vi "Neutral_ScanAgilentTrim_20151209.vi"(8 "error in (no error)":errorcluster={"status"=FALSE, "code"=0, "source"="gettemp.vi: No error - function call successful"}, 9 "Control Reference Cluster Input":T3, 11 "Triggered Voltage Settings":T1={"Trigger \nDelay (s)"=0.0, "Enable +6V Channel"=FALSE, "+6V Current"=1.0, "Enable -25V Channel"=FALSE, "-25V Current"=0.0, "Enable +25V Channel"=FALSE, "+25V Current"=0.0, "Agilent Rewrite each Cycle"=FALSE} {"Trigger \nDelay (s)" min=0.0 max=3600.0 step=1.0 format="%.2f"}) -> (0 "Error Out":errorcluster)   [LabVIEW 2016]
uses:
  Controls/Agilent E3631A/Settings_Control.ctl
  Controls/Agilent E3631A/Trigger_Settings.ctl
panel:
  in  "Agilent E3631A Settings":T2={"VISA resource name"="GPIB0::5::INSTR", "Voltage Set (6V max)"=6.0, "Current Set (5A max)"=0.007, "Voltage Set (25V max)"=25.0, "Current Set (1A max)"=0.225, "Voltage Set (-25V max)"=25.0, "Current Set (1A max)"=0.225, "6V Switch"=FALSE, "+25V Switch"=FALSE, "-25V Switch"=FALSE} {"Current Set (1A max)" format="%.3g"; "Voltage Set (-25V max)" format="%.3g"; "Current Set (1A max)" format="%.3g"; "Voltage Set (25V max)" format="%.3g"; "Current Set (5A max)" format="%.3g"; "Voltage Set (6V max)" format="%.3g"}
  # "I am assuming here that we will leave the voltage at the maximum and set set the trim field by the current limit. Assuming this will use the voltage settings from the inital programming and only vary the current limit."
  # "-25V Output Settings"
  # "+25V Output Settings"
  # "6V Output Settings"
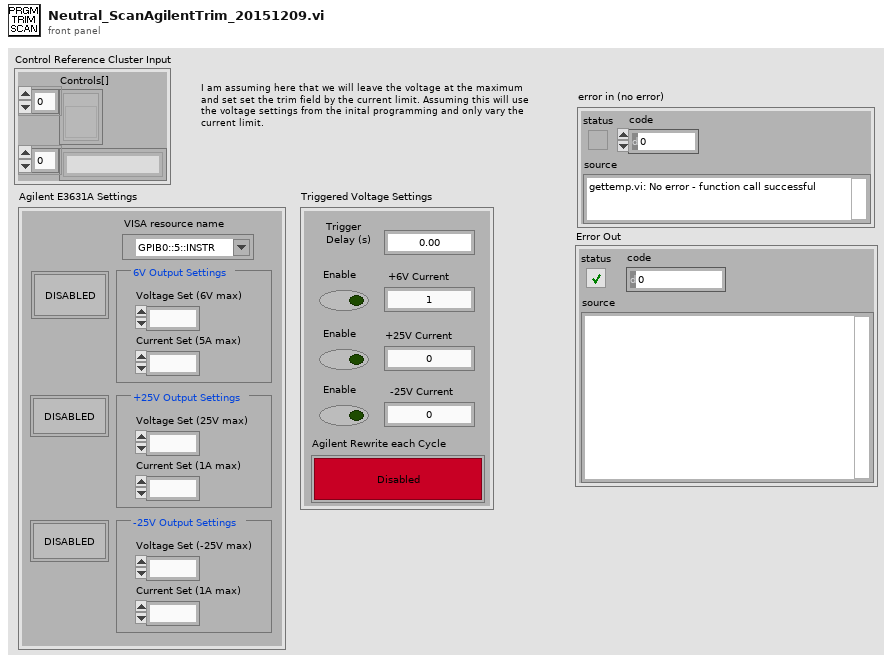
[diagram p1: front panel]
types:
  T1 = typedef "Trigger_Settings.ctl" = cluster{"Trigger \nDelay (s)":dbl, "Enable +6V Channel":bool, "+6V Current":dbl, "Enable -25V Channel":bool, "-25V Current":dbl, "Enable +25V Channel":bool, "+25V Current":dbl, "Agilent Rewrite each Cycle":bool}
  T2 = typedef "Settings_Control.ctl" = cluster{"VISA resource name":refnum<visa-resource-name>, "Voltage Set (6V max)":dbl, "Current Set (5A max)":dbl, "Voltage Set (25V max)":dbl, "Current Set (1A max)":dbl, "Voltage Set (-25V max)":dbl, "Current Set (1A max)":dbl, "6V Switch":bool, "+25V Switch":bool, "-25V Switch":bool}
  T3 = cluster{"Controls[]":refnum<vi>[], "Control Names":string[]}
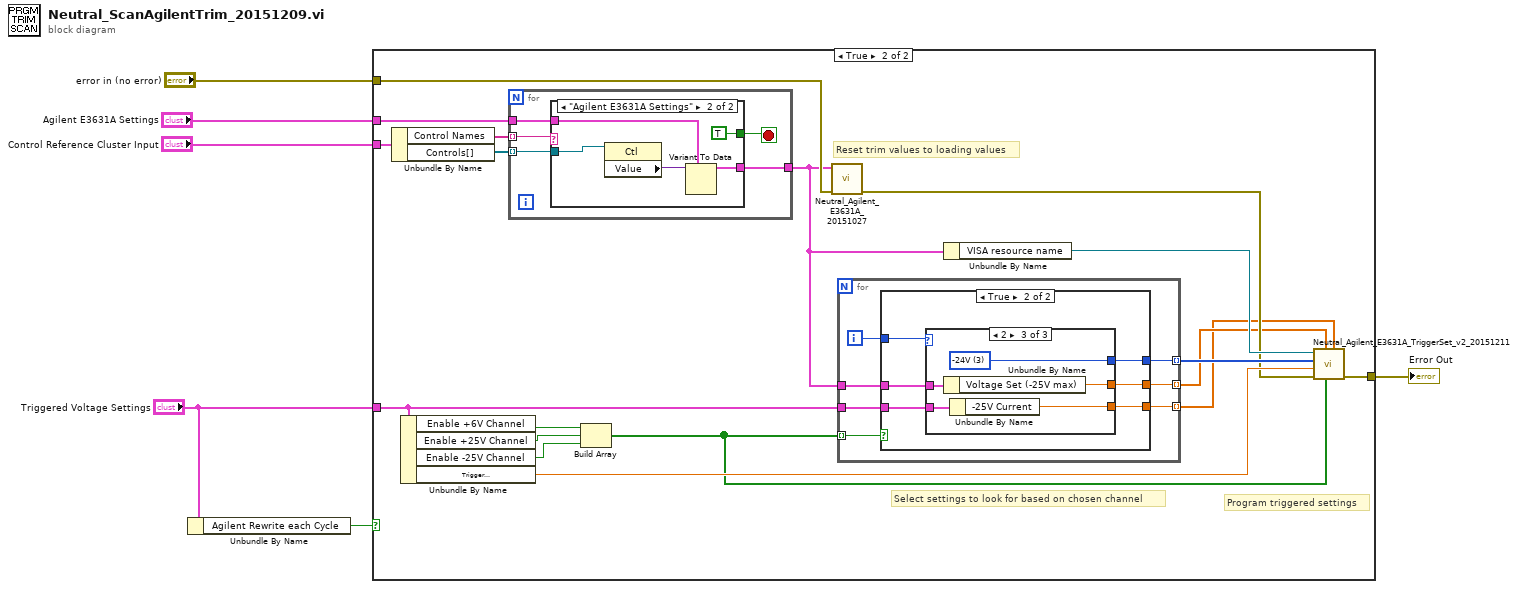
[diagram p0: block diagram]
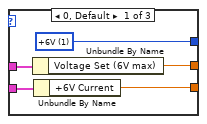
[diagram p4: hidden frame]
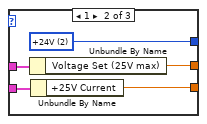
[diagram p5: hidden frame]
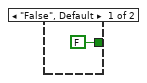
[diagram p6: hidden frame]
diagram:
  n1 = Unbundle By Name("Triggered Voltage Settings") -> ("Agilent Rewrite each Cycle"=w5:bool)
  n2 = case shown="True" w5 {
    tunnel: "Control Reference Cluster Input" -> [_ w25]
    tunnel: "Agilent E3631A Settings" -> [_ w22]
    tunnel: "Triggered Voltage Settings" -> [_ w18]
    tunnel: "error in (no error)" -> [w7 w10]
    tunnel: [w7 w9] -> w3
    frame False {
    }
    frame True {
      # "Program triggered settings"
      # "Select settings to look for based on chosen channel"
      # "Reset trim values to loading values"
      n3 = Unbundle By Name(w25) -> ("Control Names"=w24:string[], "Controls[]"=w23:refnum<vi>[])
      n4 = Unbundle By Name(w18) -> ("Enable +6V Channel"=w21:bool, "Enable +25V Channel"=w20:bool, "Enable -25V Channel"=w19:bool, "Trigger \nDelay (s)"=w15:dbl)
      n5 = for {
        tunnel: w24 -> [w58] mode=indexing
        tunnel: w23 -> [w57] mode=indexing
        tunnel: w22 -> [w56]
        tunnel: [w55] -> w8
        stop <- w54 stop-if-true
        n6 = case shown="\"Agilent E3631A Settings\"" w58 {
          tunnel: w57 -> [_ w64]
          tunnel: w56 -> [_ w62]
          tunnel: [_ w61] -> w55
          tunnel: [FALSE TRUE] -> w54
          frame "False", Default {
          }
          frame "Agilent E3631A Settings" {
            n7 = property class="Ctl"(reference=w64) -> ("Value"=w63:variant)  [unwired: 1 in, 2 out]
            n8 = Variant To Data(type=w62, Variant=w63) -> (data=w61:T2)  [unwired: 1 in, 1 out]
          }
        }
      }
      n9 = Build Array(w21, w20, w19) -> (w11:bool[])
      n10 = call "Neutral_Agilent_E3631A_20151027.vi"("error in (no error)"=w10, "Agilent E3631A Settings"=w8) -> ("error out"=w14:errorcluster)  [unwired: 8 in, 1 out]
      n11 = for {
        tunnel: [w31] -> w12 mode=indexing
        tunnel: [w30] -> w16 mode=indexing
        tunnel: w11 -> [w29] mode=indexing
        tunnel: w18 -> [w28]
        tunnel: w8 -> [w27]
        tunnel: [w26] -> w13 mode=indexing
        i -> [w32]
        n12 = case shown="True" w29 {
          tunnel: w32 -> [_ w38]
          tunnel: [_ w37] -> w31
          tunnel: [_ w36] -> w30
          tunnel: w28 -> [_ w35]
          tunnel: w27 -> [_ w34]
          tunnel: [_ w33] -> w26
          frame False {
          }
          frame True {
            n13 = case shown="2" w38 {
              tunnel: [w43 w48 w53] -> w37
              tunnel: [w42 w47 w52] -> w36
              tunnel: w35 -> [w41 w46 w51]
              tunnel: w34 -> [w40 w45 w50]
              tunnel: [w39 w44 w49] -> w33
              frame 0, Default {
                w42 = 1 items=["+6V"=1, "+24V"=2, "-24V"=3] ("Channel")
                n14 = Unbundle By Name(w40) -> ("Voltage Set (6V max)"=w39:dbl)
                n15 = Unbundle By Name(w41) -> ("+6V Current"=w43:dbl)
              }
              frame 1 {
                w47 = 2 items=["+6V"=1, "+24V"=2, "-24V"=3] ("Channel")
                n16 = Unbundle By Name(w45) -> ("Voltage Set (25V max)"=w44:dbl)
                n17 = Unbundle By Name(w46) -> ("+25V Current"=w48:dbl)
              }
              frame 2 {
                w52 = 3 items=["+6V"=1, "+24V"=2, "-24V"=3] ("Channel")
                n18 = Unbundle By Name(w50) -> ("Voltage Set (-25V max)"=w49:dbl)
                n19 = Unbundle By Name(w51) -> ("-25V Current"=w53:dbl)
              }
            }
          }
        }
      }
      n20 = Unbundle By Name(w8) -> ("VISA resource name"=w17:refnum<visa-resource-name>)
      n21 = call "Neutral_Agilent_E3631A_TriggerSet_v2_20151211.vi"("Triggeed Current Limit"=w12, "Program Trigger?"=w11, "Triggerd Voltage Level"=w13, "error in (no error)"=w14, "Trigger Delay (s)"=w15, "Channel"=w16, "VISA resource name"=w17) -> ("error out"=w9:errorcluster)  [unwired: 4 in]
    }
  }
  "Error Out" <- w3
